vi "JKISM++ Module Status.vi"(8 "Error in":errorcluster caption="Error in (no error)", 11 "JKISM Name":string) -> (0 "Error out":errorcluster, 1 "#AsWorker":i32, 2 "Mode":T1, 3 "JKISM Name(dup)":string, 4 "#msg to be processed":i32)   [LabVIEW 2014, in "JKI-State-Machine-Plus.lvlib"]
doc: "Get the JKISM+ Module Status"
uses:
  JKI-State-Machine-Plus.lvlib
  _Support/Typedef/_JKISM_MODE.ctl
  _Support/JKISMQ/_JKISMQFGVOPER.ctl
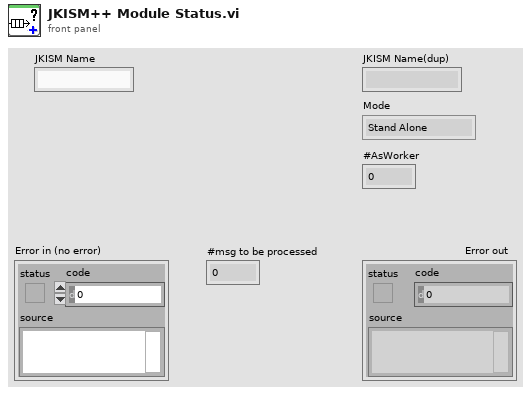
[diagram p1: front panel]
types:
  T1 = typedef "JKI-State-Machine-Plus.lvlib/_JKISM_MODE.ctl" = enum16{"Stand Alone", "JKISM", "Action Worker"}
  T2 = typedef "JKI-State-Machine-Plus.lvlib/_JKISMQFGVOPER.ctl" = enum16{"Get By Name", "List", "Check If Name Exists", "Release", "Module Status"}
  T3 = typedef "JKI-State-Machine-Plus.lvlib/_JKISMQ.ctl" = cluster{"Module Name":string, "Queue":refnum<queue>, "Locked Status":refnum<data-value>, "Mode":T1, "UserEvent":refnum<user-event>, "Queue Count":i32}
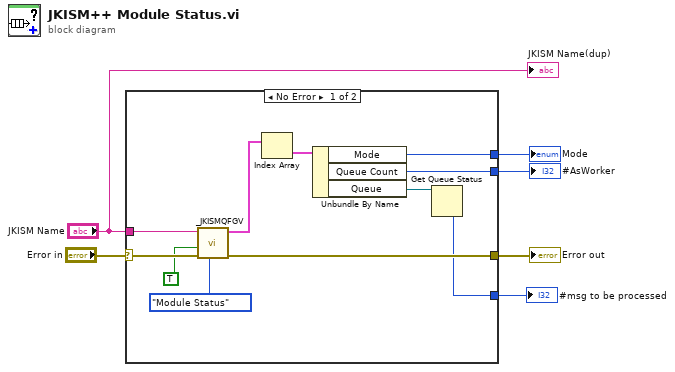
[diagram p0: block diagram]
diagram:
  n1 = case shown="No Error" "Error in" {
    selector: "Error in" -> [w17 w18]
    tunnel: [w16 w18] -> w5
    tunnel: [w11 _] -> w4
    tunnel: [w10 _] -> w3
    tunnel: [w8 _] -> w2
    tunnel: "JKISM Name" -> [w7 _]
    frame No Error {
      n2 = call "_JKISMQFGV.vi"(6:_JKISMQFGVOPER."Module Status", "Error in"=w17, "create if not found? (T)"=TRUE ("Exclude Standalone JKISM(T)"), "Name(\"\" to use uuid) in"=w7) -> ("Error out"=w16:errorcluster, "Array"=w13:T3[])  [unwired: 4 in, 2 out]
      n3 = Index Array(array=w13) -> (element=w12:T3)  [unwired: 1 in]
      n4 = Unbundle By Name(w12) -> ("Mode"=w11:T1, "Queue Count"=w10:i32, "Queue"=w9:refnum<queue>)
      n5 = Get Queue Status(queue=w9) -> (# elements in queue=w8:i32)  [unwired: 2 in, 7 out]
    }
    frame Error {
    }
  }
  "Error out" <- w5
  "Mode" <- w4
  "#AsWorker" <- w3
  "#msg to be processed" <- w2
  "JKISM Name(dup)" <- "JKISM Name"
